vi "DDE Poke.vi"(5 "timeout (-1)":i32=-1, 6 "error in (no error)":errorcluster, 7 "data":string, 8 "item":string, 9 "conversation refnum in":u32) -> (0 "error out":errorcluster, 3 "conversation refnum out":u32)   [LabVIEW 2014]
doc: "Pokes data to a location. Refer to the Using DDE in LabVIEW Application Note for more information about DDE.\n\n<B>timeout</B> indicates how many milliseconds to wait for the function to complete. The default is -1, which indicates no timeout. If the VI completes before the specified amount of time, it returns an error.\n\n<B>conversation refnum</B> is a refnum that uniquely identifies this DDE conversation.\n\n<B>item</B> is the location where the VI pokes the <B>data</B>.\n\n<B>data</B> contains the data the VI sends.\n\n<B>error in</B> describes error conditions that occur before this VI or function runs. The default is no error. If an error occurred before this VI or function runs, the VI or function passes the <B>error in</B> value to <B>error out</B>. This VI or function runs normally only if no error occurs before this VI or function runs. If an error occurs while this VI or function runs, it runs normally and sets its own error status in <B>error out</B>. Use the Simple Error Handler or General Error Handler VIs to display the description of the error code. Use <B>error in</B> and <B>error out</B> to check errors and to specify execution order by wiring <B>error out</B> from one node to <B>error in</B> of the next node.\n\n<B>status</B> is TRUE (X) if an error occurred before this VI or function ran or FALSE (checkmark) to indicate a warning or that no error occurred before this VI or function ran. The default is FALSE.\n\n<B>code</B> is the error or warning code. The default is 0.\nIf <B>status</B> is TRUE, <B>code</B> is a non-zero error code. If <B>status</B> is FALSE, <B>code</B> is 0 or a warning code.\n\n<B>source</B> describes the origin of the error or warning and is, in most cases, the name of the VI or function that produced the error or warning. The default is an empty string.\n\n<B>conversation refnum</B> is a refnum that uniquely identifies this DDE conversation. It passes through this VI to assist in execution timing.\n\n<B>error out</B> contains error information. If <B>error in</B> indicates that an error occurred before this VI or function ran, <B>error out</B> contains the same error information. Otherwise, it describes the error status that this VI or function produces. Right-click the <B>error out</B> indicator on the front panel and select <B>Explain Error</B> from the shortcut menu for more information about the error.\n\n<B>status</B> is TRUE (X) if an error occurred or FALSE (checkmark) to indicate a warning or that no error occurred.\n\n<B>code</B> is the error or warning code. If <B>status</B> is TRUE, <B>code</B> is a non-zero error code. If <B>status</B> is FALSE, <B>code</B> is 0 or a warning code.\n\n<B>source</B> describes the origin of the error or warning and is, in most cases, the name of the VI or function that produced the error or warning."
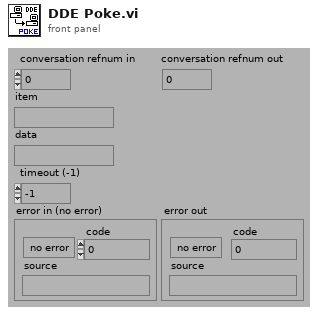
[diagram p1: front panel]
types:
  T1 = cluster{i8, u32[], "item":string, "data":string, bool}
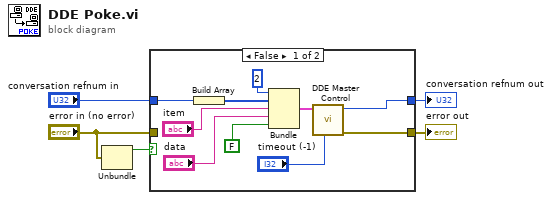
[diagram p0: block diagram]
diagram:
  n1 = Unbundle("error in (no error)") -> ("status"=w3:bool)  [unwired: 2 out]
  n2 = case shown="False" w3 {
    tunnel: [w11 w17] -> w1
    tunnel: [w9 w16] -> w5
    tunnel: "error in (no error)" -> [_ w17]
    tunnel: "conversation refnum in" -> [w10 w16]
    frame False {
      n3 = Build Array(w10) -> (w6:u32[])
      n4 = Bundle(i8 2, w6, "item"="item", "data"="data", FALSE) -> (w12:T1)  [unwired: 1 in]
      n5 = call "DDE Master Control.vi"("timeout(-1)"="timeout (-1)", "input"=w12) -> ("error out"=w11:errorcluster, "refnum"=w9:u32)  [unwired: 3 in, 3 out]
    }
    frame True {
    }
  }
  "conversation refnum out" <- w5
  "error out" <- w1
